vi "Process 4 Page.vi"() -> ()   [LabVIEW 2019]
uses:
  <vilib>/NI/Current Value Table/Type Defs/Single Tag.ctl
  <vilib>/NI/Current Value Table/Type Defs/Data Types.ctl
  <vilib>/NI/STM/TCP/Read Meta Data (TCP Ref).vi
  <vilib>/NI/STM/TCP/Get Connection Reference (TCP).vi
  <vilib>/NI/AMC/Read Termination Message.vi
  <vilib>/NI/AMC/Create Single Message.vi
  <vilib>/NI/AMC/Update Message Routing Info.vi
  <vilib>/NI/STM/TCP/Read Meta Data (TCP Clst).vi
  <vilib>/NI/AMC/Globals.vi
  <vilib>/NI/STM/TCP/Write Message (TCP).vi
  <vilib>/NI/AMC/Send Message.vi
  <vilib>/NI/AMC/AMC.lvlib
  <vilib>/NI/STM/NI STM.lvlib
  <vilib>/NI/Current Value Table/Current Value Table.lvlib
panel:
  in  "Sulfuric Add Volume":dbl min=0.0 max=500.0 step=0.25
  in  "Add Sulfuric":bool
  out "Di Add Pipe 2":bool
  out "Di Water Elbow 2":bool
  out "Liters DI Added 2":dbl caption="Liters Sulfuric Added" format="%.1f"
  out "Sulfuric Flow Rate":dbl(knob) scale=0.0..75.0
  out "Boolean 6":bool
  out "Boolean 5":bool
  in  "Pump Speed 4":dbl=5.0 caption="Pump Speed" min=5.0 max=100.0 step=0.5
  out "RPM":dbl(knob) scale=0.0..3500.0
  out "DI Flow Rate":dbl(knob) scale=0.0..75.0
  out "SG":dbl format="%.4g"
  in  "Bath SG":dbl=1.8 min=0.9 max=1.8 step=0.0025 format="%.4g"
  out "Recirc Elbow":bool
  out "Di Add Pipe":bool
  out "Di Water Elbow":bool
  out "Liters DI Added 1":dbl caption="Liters DI Added" format="%.1f"
  in  "DI Add Volume 1":dbl caption="DI Add Volume" min=0.0 max=500.0 step=0.25
  in  "Add DI water 1":bool caption="Add DI Water"
  in  "Drain System to Tree 1":bool caption="Drain System to Tree"
  in  "Enable Main Pump":bool
  out "Sump Return":bool
  out "PipeFromPmp":bool
  out "Proc4MainPumpInd 2":bool
  out "Tank 2":dbl(slide) caption="Tank" scale=0.0..1000.0
  out "Run Enabled":bool
  in  "Dosing":bool
  in  "Mixing Tank":bool
  in  "Process 3":bool
  in  "Process 2":bool
  in  "Process 1":bool
  out "status":string
  in  "Home Btn":bool
  in  "Facilities Btn":bool
  # "%"
  # "T 340"
  # "L"
  # "@"
  # "L"
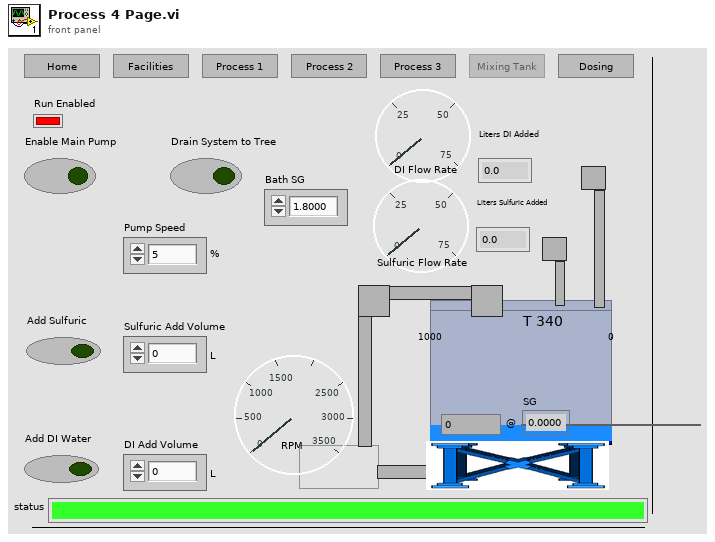
[diagram p1: front panel]
types:
  T1 = typedef "Current Value Table.lvlib/Single Tag.ctl" = cluster{"Data Type":T2, "Name":string, "Value":string, "Description":string}
  T2 = typedef "Current Value Table.lvlib/Data Types.ctl" = enum16{"Double", "Single", "I64", "I32", "I16", "I8", "U64", "U32", "U16", "U8", "String", "Boolean", "Array of U8", "Array of U16", "Array of U32", "Array of U64", "Array of I64", "Array of I32", "Array of I16", "Array of I8", "Array of Double", "Array of Single", "Array of Boolean", "Array of String"}
  T3 = typedef "AMC.lvlib/Message Queue.ctl" = refnum<queue>
  T4 = typedef "NI STM.lvlib/TCP Connection Info.ctl" = cluster{"connection ID":refnum<k5>, "meta data":T5[]}
  T5 = typedef "NI STM.lvlib/MetaDataElement.ctl" = string
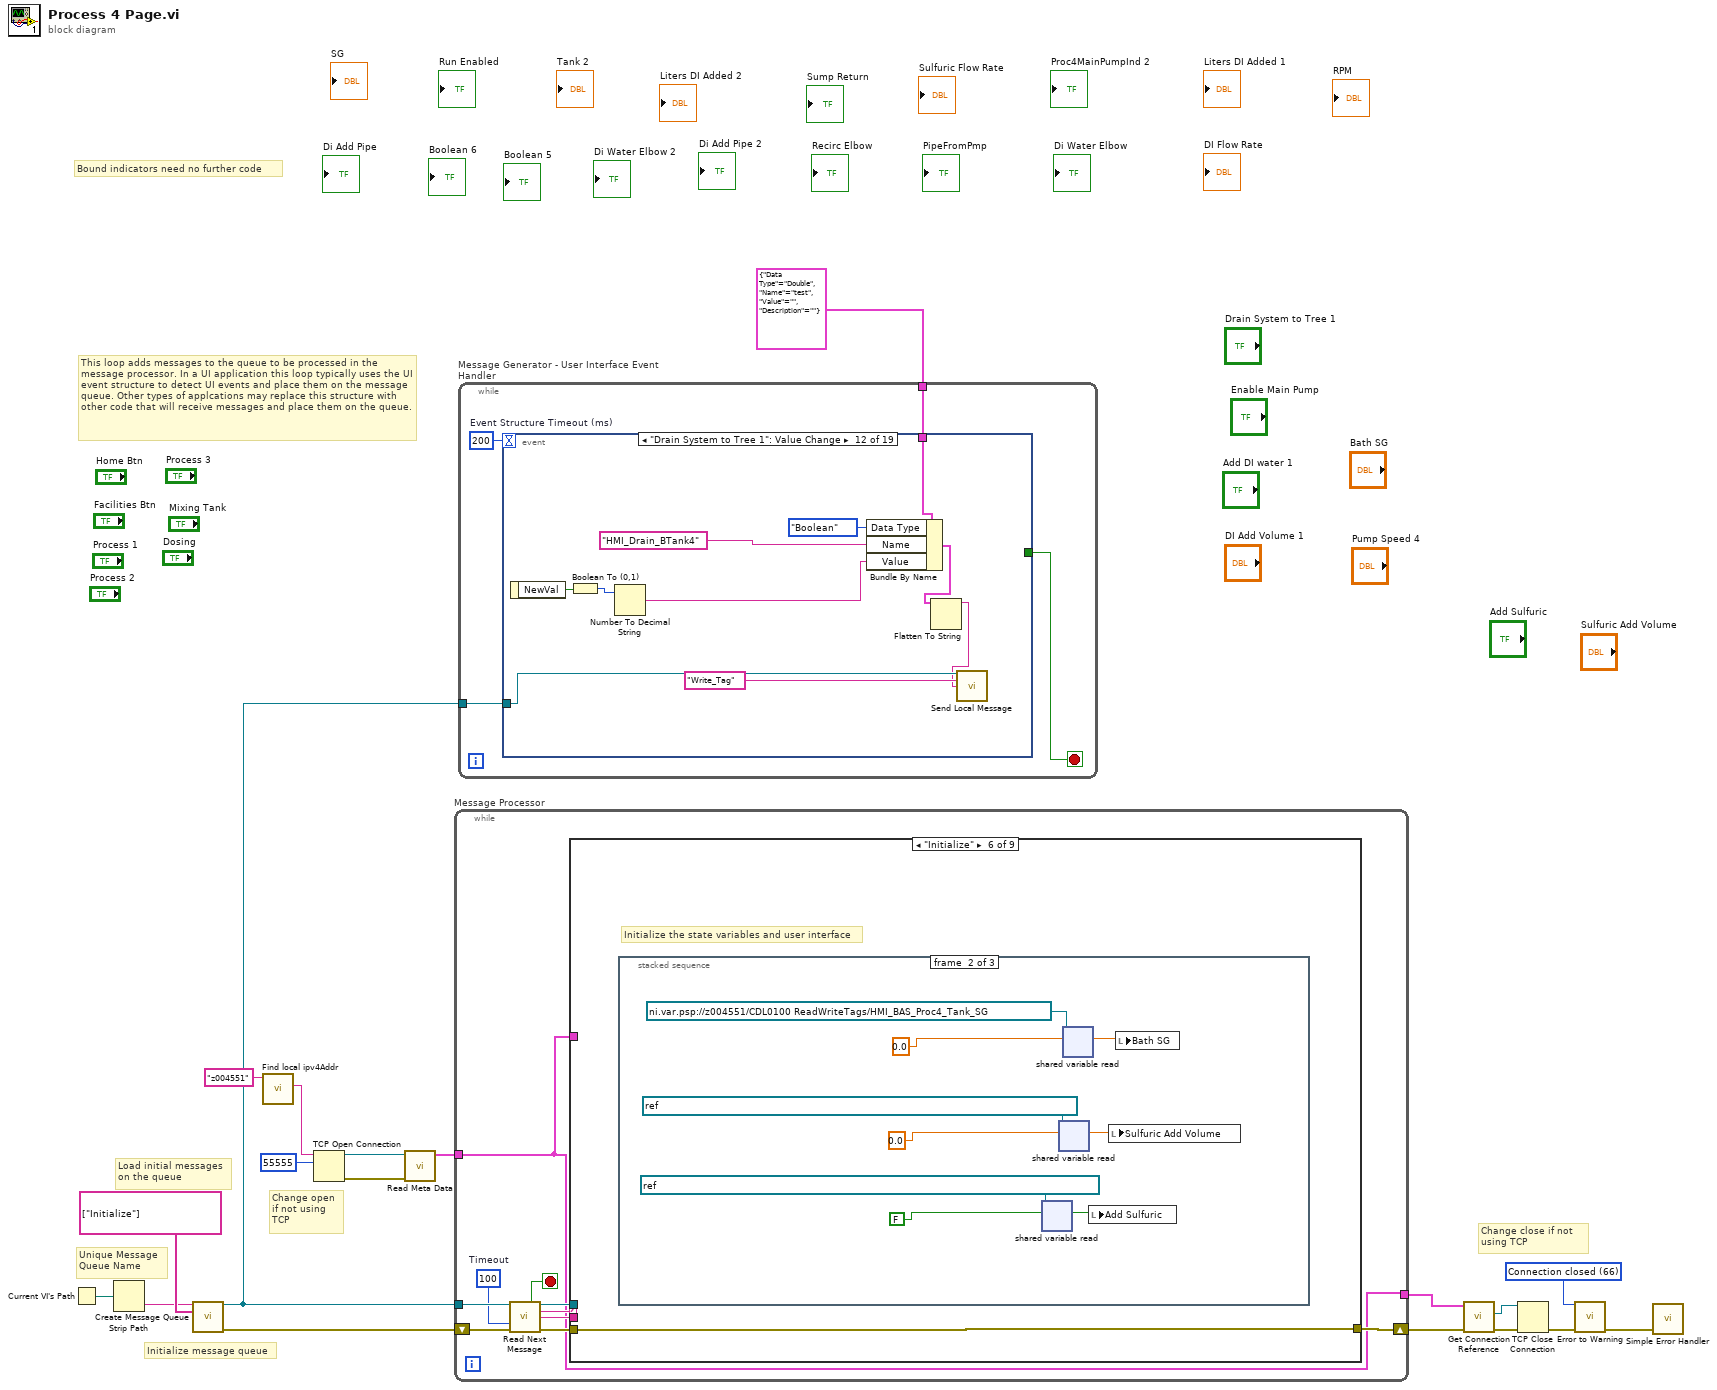
[diagram p0: block diagram]
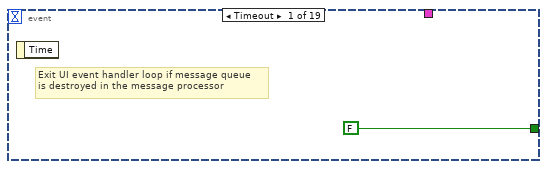
[diagram p2: hidden frame]
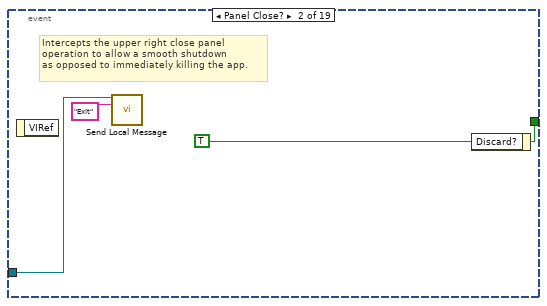
[diagram p3: hidden frame]
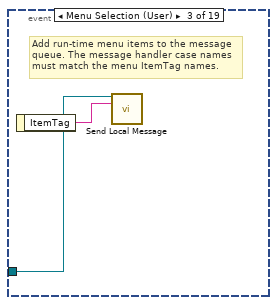
[diagram p4: hidden frame]
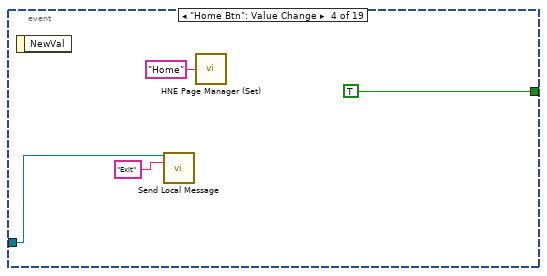
[diagram p5: hidden frame]
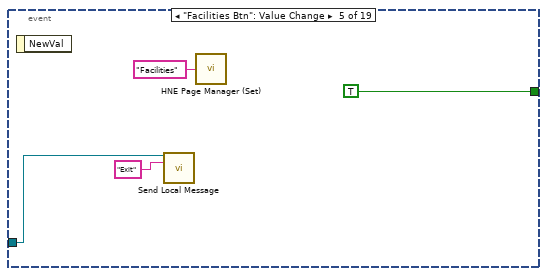
[diagram p6: hidden frame]
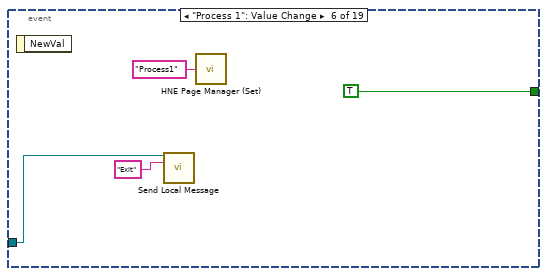
[diagram p7: hidden frame]
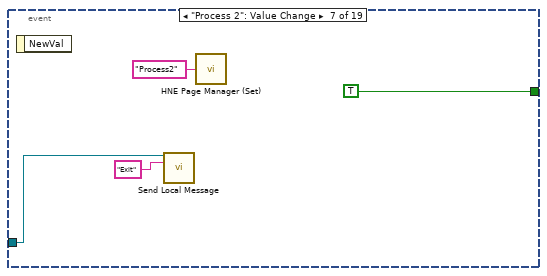
[diagram p8: hidden frame]
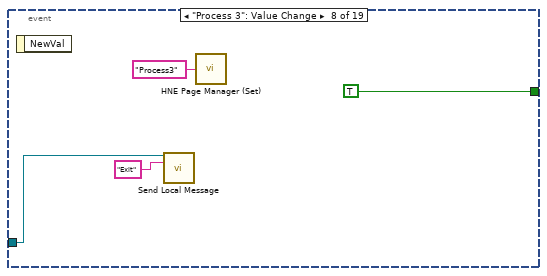
[diagram p9: hidden frame]
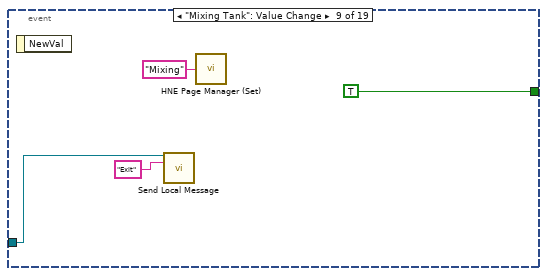
[diagram p10: hidden frame]
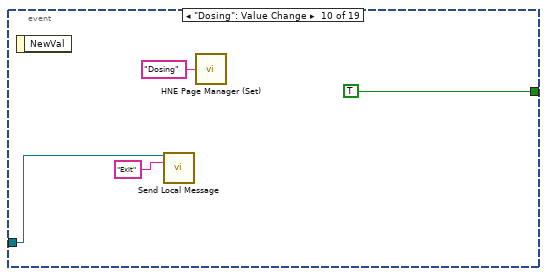
[diagram p11: hidden frame]
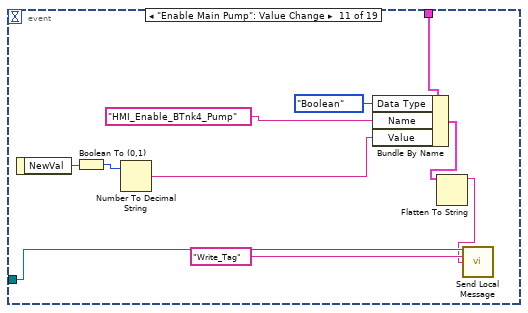
[diagram p12: hidden frame]
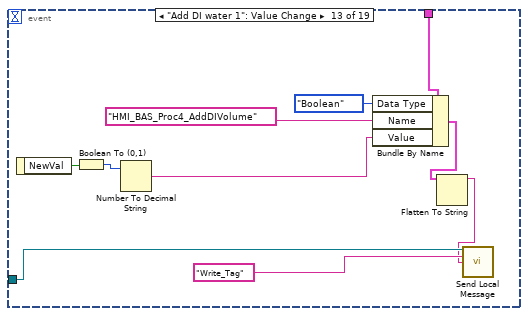
[diagram p13: hidden frame]
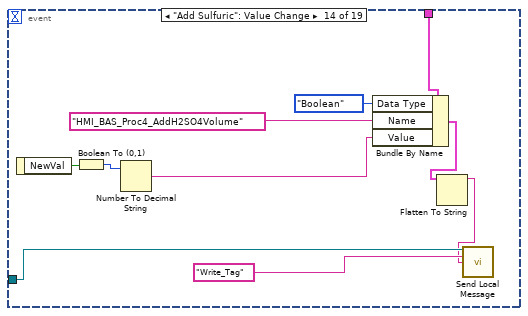
[diagram p14: hidden frame]
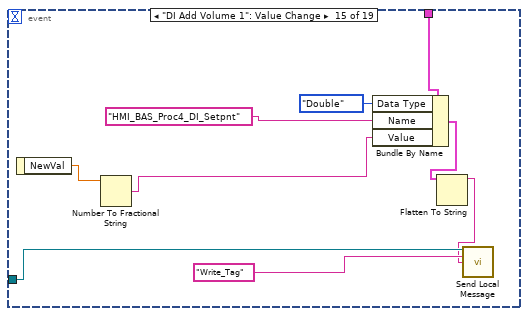
[diagram p15: hidden frame]
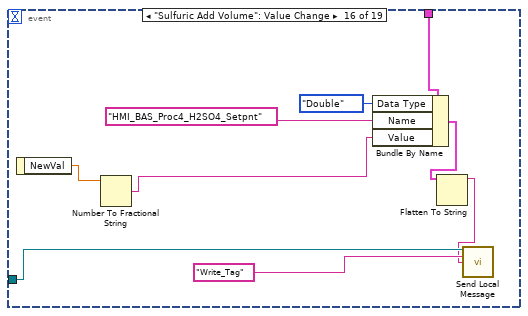
[diagram p16: hidden frame]
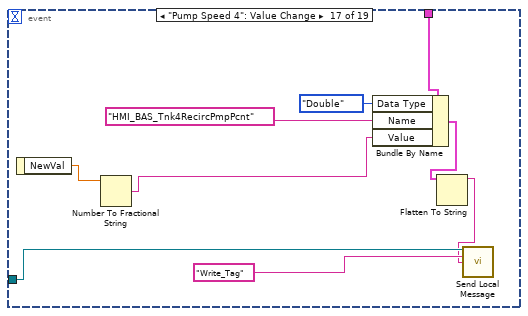
[diagram p17: hidden frame]
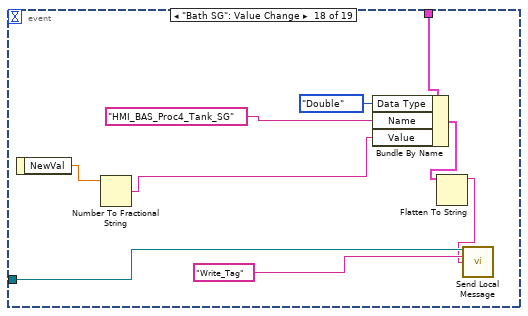
[diagram p18: hidden frame]
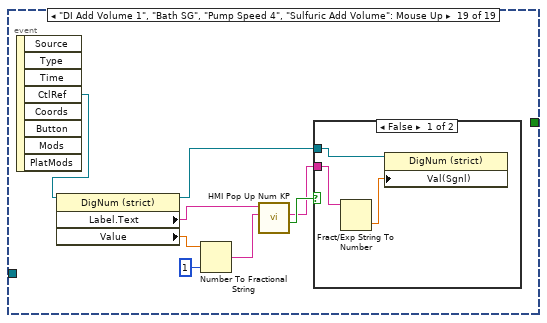
[diagram p19: hidden frame]
diagram:
  w8 = 66 items=["No Error", "Argument Error", "Memory Full", "Out of Zone", "End of File", "File Already Open", "Generic File IO Error", "File Not Found", "File Permission Error", "Disk Full", "Duplicate Path", "Too Many Files Open", "Not Enabled", "Resource File Not Found", "Cannot Add Resource", "Resource Not Found", "Image Not Found", "Image Memory Error", "Pen Does Not Exist", "Config Bad Type", "Config Token Not Found", "Config Parse Error", "Config Memory Error", "Bad External Code Format", "Bad External Code Offset", "External Code Not Present", "Null Window", "Destroy Window Mixup", "Null Menu", "Print Aborted", "Bad Print Record", "Print Driver Error", "Windows Error During Print", "Memory Error During Print", "Print Dialog Error", "Generic Print Error", "Invalid Device Refnum", "Device Not Found", "Device Parameter Error", "Device Unit Error", "Can't Open Device", "Device Call Aborted", "Generic Error", "Cancelled By User", "Object ID Too Low", "Object ID Too High", "Object Not In Heap", "Unknown Heap", "Bad DefProc ID", "DefProc Not In Table", "Message Out Of Range", "Null Method", "Unknown Message", "Manager Call Not Supported", "Bad address", "Connection In progress", "Connection timed out", "Connection is already in progress", "Network attribute not supported", "Network error", "Address in use", "System out of memory", "Connection aborted", "Connection refused", "Connection is not connected", "Connection is already connected", "Connection closed", "Initialize error (interapplication manager)", "Bad occurrence", "Wait on unbound occurrence handler", "Occurrence queue overflow", "Bad path", "Semaphore not signaled", "Unrecognized type (interapplication manager)"] ("1st Error to Convert")
  # "Bound indicators need no further code"
  # "Change close if not using TCP"
  # "Change open if not using TCP"
  # "This loop adds messages to the queue to be processed in the message processor. In a UI application this loop typically uses the UI event structure to detect UI events and place them on the message queue. Other types of applcations may replace this structure with other code that will receive messages and place them on the queue."
  # "Initialize message queue"
  # "Unique Message\nQueue Name"
  # "Load initial messages\non the queue"
  n1 = Current VI's Path() -> (path=w15:path)
  n2 = Strip Path(path=w15) -> (name=w18:string)  [unwired: 1 out]
  n3 = call <vilib>:"Create Message Queue.vi"("message queue name"=w18, "initial message names"=string[] ["Initialize"]) -> ("message queue out"=w17:T3, "error out"=w16:errorcluster)  [unwired: 12 in]
  n4 = call "Find local ipv4Addr.vi"("MachineToFind"="z004551") -> ("name"=w11:string)  [unwired: 9 in, 1 out]
  n5 = TCP Open Connection(address=w11, remote port or service name=u16 55555 ("remote port")) -> (connection ID=w13:refnum<k5>, error out=w12:errorcluster)  [unwired: 1 in, 2 out]
  n6 = call-poly <vilib>:"Read Meta Data.vi"("error in"=w12, "connection ID"=w13) -> ("connection info out"=w3:T4)  [unwired: 7 in, 2 out]
  n7 = while "Message Processor" {
    shift-left: w16 -> [w25]
    shift-right: [w29] -> w4
    tunnel: w17 -> [w26]
    tunnel: [w20] -> w2
    tunnel: w3 -> [w20]
    stop <- w28 stop-if-true
    w21 = 100  # Timeout
    n8 = call <vilib>:"Read Next Message.vi"("message queue in"=w26, "timeout (1 ms)"=w21, "error in"=w25) -> ("exit process?"=w28:bool, "message queue out"=w27:T3, "message name"=w23:string, "message value"=w22:string, "error out"=w24:errorcluster)  [unwired: 5 in, 3 out]
    n9 = case shown="\"Initialize\"" w23 {
      selector: w23 -> [_ _ w56 _ _ _ _ _ _]
      tunnel: w27 -> [_ _ _ _ _ _ w90 _ _]
      tunnel: w24 -> [w30 w32 w57 w58 w60 w61 w91 w93 w95]
      tunnel: [w30 w32 w57 errorcluster {"status"=FALSE, "code"=0, "source"=""} ("error out") w60 w61 w89 w93 w94] -> w29
      tunnel: w22 -> [_ _ _ _ _ _ _ _ w96]
      tunnel: w20 -> [_ _ _ _ _ _ _ _ w97]
      frame "---------- Framework Operations ----------" {
        # "Dummy case to add a seperator in the Case Structure menu"
      }
      frame "", "Idle" {
        # "Idle Case - this case is called after a Timeout on the Get Next Message from Queue VI, if no new messages are present on the queue. This case can be used for housekeeping tasks such as updating the UI."
        n10 = stacked-sequence {
          frame #0 {
            # "Other HMI changed state - align"
            n11 = shared-variable-read(refnum<k21> "ni.var.psp://z004551/CDL0100 ReadWriteTags/HMI_Enable_BTnk4_Pump" ("shared variable refnum in"), FALSE ("data type")) -> (w33:bool)  [unwired: 1 in, 3 out]
            n12 = call <userlib>:"Boolean Trigger__ogtk.vi"("Boolean Input"=w33) -> ("Rising Edge"=w38:bool, "Falling Edge"=w37:bool)  [unwired: 1 in]
            n13 = Or(x=w38, y=w37) -> (x .or. y?=w36:bool)
            n14 = case shown="True" w36 {
              tunnel: w33 -> [_ w39]
              frame False {
              }
              frame True {
                n15 = local write "Enable Main Pump"(w39) -> ()
              }
            }
          }
          frame #1 {
            n16 = shared-variable-read(refnum<k21> "ni.var.psp://z004551/CDL0100 ReadWriteTags/HMI_BAS_Proc4_AddDIVolume" ("shared variable refnum in"), FALSE) -> (w45:bool)  [unwired: 1 in, 3 out]
            n17 = shared-variable-read(refnum<k21> "ni.var.psp://z004551/CDL0100 ReadWriteTags/HMI_BAS_Proc4_AddH2SO4Volume" ("shared variable refnum in"), FALSE) -> (w41:bool)  [unwired: 1 in, 3 out]
            n18 = call <userlib>:"Boolean Trigger__ogtk.vi"("Boolean Input"=w45) -> ("Falling Edge"=w44:bool)  [unwired: 1 in, 1 out]
            n19 = call <userlib>:"Boolean Trigger__ogtk.vi"("Boolean Input"=w41) -> ("Falling Edge"=w40:bool)  [unwired: 1 in, 1 out]
            n20 = case shown="True" w40 {
              frame False {
              }
              frame True {
                n21 = local write "Add Sulfuric"(FALSE) -> ()
              }
            }
            n22 = case shown="True" w44 {
              frame False {
              }
              frame True {
                n23 = local write "Add DI water 1"(FALSE) -> ()
              }
            }
          }
          frame #2 {
            n24 = control-ref of="Enable Main Pump"() -> (w50:refnum<vi>)
            n25 = control-ref of="Drain System to Tree 1"() -> (w52:refnum<vi>)
            n26 = call "GrayOutButtonFromPSPVar.vi"("shared variable refnum in"=refnum<k21> "ni.var.psp://z004551/CDL0100 ReadWriteTags/HMI_Drain_BTank4", "Boolean in"=w50) -> ()  [unwired: 10 in]
            n27 = call "GrayOutButtonFromPSPVar.vi"("shared variable refnum in"=refnum<k21> "ni.var.psp://z004551/CDL0100 ReadWriteTags/HMI_Enable_BTnk4_Pump", "Boolean in"=w52) -> ()  [unwired: 10 in]
          }
        }
        n28 = control-ref of="status"() -> (w31:refnum<vi>)
        n29 = call <userlib>:"TAE Format Alarm Ticker.vi"("Alarm Ticker Ref"=w31) -> ()  [unwired: 15 in]
      }
      frame "Missing Message Handler", Default {
        # "Call this case if a message is received that is not handled \nby any other case. Typically this is a programming error\nas a result of a typo or unhandled message/missing message handler."
        n30 = Format Into String(format string="DevError: Missing message handler for '%s\" message." ("message"), w56) -> (resulting string=w54:string)  [unwired: 2 in, 1 out]
        n31 = One Button Dialog(message=w54) -> ()  [unwired: 2 out]
      }
      frame "Error" {
        # "General Error Case - this case is called if an error is passed using the error cluster below. Typically most new errors should be handed in each individual case and not passed in the rror cluster. If necessary a custom error handler case should be added and called from other cases."
        n32 = call <vilib>:"Simple Error Handler.vi"("error in (no error)"=w58) -> ()  [unwired: 1 in, 8 out]
      }
      frame "---------- Generic Operations ----------" {
        # "Dummy case to add a seperator in the Case Structure menu"
      }
      frame "Initialize" {
        # "Initialize the state variables and user interface"
        n33 = stacked-sequence {
          frame #0 {
            n34 = shared-variable-read(refnum<k21> "ni.var.psp://z004551/CDL0100 ReadWriteTags/HMI_Drain_BTank4" ("shared variable refnum in"), FALSE) -> (w68:bool)  [unwired: 1 in, 3 out]
            n35 = shared-variable-read(refnum<k21> "ni.var.psp://z004551/CDL0100 ReadWriteTags/HMI_BAS_Proc4_AddDIVolume" ("shared variable refnum in"), FALSE) -> (w65:bool)  [unwired: 1 in, 3 out]
            n36 = shared-variable-read(refnum<k21> "ni.var.psp://z004551/CDL0100 ReadWriteTags/HMI_Enable_BTnk4_Pump" ("shared variable refnum in"), FALSE) -> (w71:bool)  [unwired: 1 in, 3 out]
            n37 = shared-variable-read(refnum<k21> "ni.var.psp://z004551/CDL0100 ReadWriteTags/HMI_BAS_Proc4_DI_Setpnt" ("shared variable refnum in"), 0.0) -> (w62:dbl)  [unwired: 1 in, 3 out]
            n38 = local write "Drain System to Tree 1"(w68) -> ()
            n39 = local write "Add DI water 1"(w65) -> ()
            n40 = local write "Enable Main Pump"(w71) -> ()
            n41 = local write "DI Add Volume 1"(w62) -> ()
          }
          frame #1 {
            n42 = shared-variable-read(refnum<k21> "ni.var.psp://z004551/CDL0100 ReadWriteTags/HMI_BAS_Proc4_AddH2SO4Volume" ("shared variable refnum in"), FALSE) -> (w74:bool)  [unwired: 1 in, 3 out]
            n43 = shared-variable-read(refnum<k21> "ni.var.psp://z004551/CDL0100 ReadWriteTags/HMI_BAS_Proc4_H2SO4_Setpnt" ("shared variable refnum in"), 0.0) -> (w77:dbl)  [unwired: 1 in, 3 out]
            n44 = shared-variable-read(refnum<k21> "ni.var.psp://z004551/CDL0100 ReadWriteTags/HMI_BAS_Proc4_Tank_SG" ("shared variable refnum in"), 0.0) -> (w80:dbl)  [unwired: 1 in, 3 out]
            n45 = local write "Add Sulfuric"(w74) -> ()
            n46 = local write "Sulfuric Add Volume"(w77) -> ()
            n47 = local write "Bath SG"(w80) -> ()
          }
          frame #2 {
            n48 = shared-variable-read(refnum<k21> "ni.var.psp://z004551/CDL0100 ReadTags/BAS_Proc4_DI_FlowRate" ("shared variable refnum in"), 0.0) -> (w86:dbl)  [unwired: 1 in, 3 out]
            n49 = shared-variable-read(refnum<k21> "ni.var.psp://z004551/CDL0100 ReadWriteTags/HMI_BAS_Tnk4RecircPmpPcnt" ("shared variable refnum in"), 0.0) -> (w83:dbl)  [unwired: 1 in, 3 out]
            n50 = local write "Pump Speed 4"(w83) -> ()
            n51 = local write "DI Flow Rate"(w86) -> ()
          }
        }
      }
      frame "Exit" {
        # "Destroy message queue >> this will halt the UI event handler loop"
        # "Stop the VI\n>> Perform any cleanup tasks in this message case.\n>> Clear display before closing."
        n52 = call <vilib>:"Destroy Message Queue.vi"("message queue in"=w90, "error in"=w91) -> ("error out"=w89:errorcluster)  [unwired: 11 in, 2 out]
        n53 = local write "status"("" ("Status")) -> ()
      }
      frame "---------- Application Operations ----------" {
        # "Dummy case to add a seperator in the Case Structure menu"
      }
      frame "Write_Tag" {
        n54 = call-poly <vilib>:"Write Message.vi"("error in"=w95, "data"=w96, "name"="WriteTag", "connection info in"=w97) -> ("error out"=w94:errorcluster)  [unwired: 6 in, 1 out]
      }
    }
  }
  n55 = while "Message Generator - User Interface Event Handler" {
    tunnel: w17 -> [w100]
    tunnel: T1 {"Data Type"=enum."Double", "Name"="test", "Value"="", "Description"=""} ("Tag") -> [w99]
    stop <- w101 stop-if-true
    w102 = 200  # Event Structure Timeout (ms)
    n56 = event shown="[11] \"Drain System to Tree 1\": Value Change" {
      selector: _ -> [_ _ _ _ _ _ _ _ _ _ _ _ _ _ _ _ _ _ _]
      dyn-events: _ -> [_ _ _ _ _ _ _ _ _ _ _ _ _ _ _ _ _ _ _]
      timeout: w102 -> [_ _ _ _ _ _ _ _ _ _ _ _ _ _ _ _ _ _ _]
      tunnel: [FALSE ("Discard?") w106 _ TRUE ("Discard?") TRUE ("Discard?") TRUE ("Discard?") TRUE ("Discard?") TRUE ("Discard?") TRUE ("Discard?") TRUE ("Discard?") _ _ _ _ _ _ _ _ _] -> w101
      tunnel: w100 -> [_ w104 w107 w109 w113 w117 w121 w125 w129 w133 w139 w149 w159 w169 w181 w190 w199 w208 _]
      tunnel: w99 -> [_ _ _ _ _ _ _ _ _ _ w144 w154 w164 w174 w185 w194 w203 w212 _]
      event Timeout {
        # "Exit UI event handler loop if message queue\nis destroyed in the message processor"
        n57 = event-data() -> ()  [unwired: 2 out]
      }
      event Panel Close? {
        w106 = TRUE ("Discard?")
        # "Intercepts the upper right close panel\noperation to allow a smooth shutdown\nas opposed to immediately killing the app."
        n58 = event-data() -> ()  [unwired: 2 out]
        n59 = call <vilib>:"Send Local Message.vi"("message queue in"=w104, "message name"="Exit") -> ()  [unwired: 11 in, 3 out]
        n60 = event-data("Discard?"=w106) -> ()  [unwired: 1 in, 1 out]
      }
      event Menu Selection (User) {
        # "Add run-time menu items to the message\nqueue. The message handler case names must match the menu ItemTag names."
        n61 = event-data() -> ("ItemTag"=w108:string)  [unwired: 1 out]
        n62 = call <vilib>:"Send Local Message.vi"("message queue in"=w107, "message name"=w108) -> ()  [unwired: 11 in, 3 out]
      }
      event "Home Btn": Value Change {
        n63 = event-data() -> ()  [unwired: 2 out]
        n64 = call <vilib>:"Send Local Message.vi"("message queue in"=w109, "message name"="Exit") -> ()  [unwired: 11 in, 3 out]
        n65 = call <userlib>:"HNE Page Manager (Set).vi"("Next Page"="Home") -> ()  [unwired: 4 in, 1 out]
      }
      event "Facilities Btn": Value Change {
        n66 = event-data() -> ()  [unwired: 2 out]
        n67 = call <vilib>:"Send Local Message.vi"("message queue in"=w113, "message name"="Exit") -> ()  [unwired: 11 in, 3 out]
        n68 = call <userlib>:"HNE Page Manager (Set).vi"("Next Page"="Facilities") -> ()  [unwired: 4 in, 1 out]
      }
      event "Process 1": Value Change {
        n69 = event-data() -> ()  [unwired: 2 out]
        n70 = call <vilib>:"Send Local Message.vi"("message queue in"=w117, "message name"="Exit") -> ()  [unwired: 11 in, 3 out]
        n71 = call <userlib>:"HNE Page Manager (Set).vi"("Next Page"="Process1") -> ()  [unwired: 4 in, 1 out]
      }
      event "Process 2": Value Change {
        n72 = event-data() -> ()  [unwired: 2 out]
        n73 = call <vilib>:"Send Local Message.vi"("message queue in"=w121, "message name"="Exit") -> ()  [unwired: 11 in, 3 out]
        n74 = call <userlib>:"HNE Page Manager (Set).vi"("Next Page"="Process2") -> ()  [unwired: 4 in, 1 out]
      }
      event "Process 3": Value Change {
        n75 = event-data() -> ()  [unwired: 2 out]
        n76 = call <vilib>:"Send Local Message.vi"("message queue in"=w125, "message name"="Exit") -> ()  [unwired: 11 in, 3 out]
        n77 = call <userlib>:"HNE Page Manager (Set).vi"("Next Page"="Process3") -> ()  [unwired: 4 in, 1 out]
      }
      event "Mixing Tank": Value Change {
        n78 = event-data() -> ()  [unwired: 2 out]
        n79 = call <vilib>:"Send Local Message.vi"("message queue in"=w129, "message name"="Exit") -> ()  [unwired: 11 in, 3 out]
        n80 = call <userlib>:"HNE Page Manager (Set).vi"("Next Page"="Mixing") -> ()  [unwired: 4 in, 1 out]
      }
      event "Dosing": Value Change {
        n81 = event-data() -> ()  [unwired: 2 out]
        n82 = call <vilib>:"Send Local Message.vi"("message queue in"=w133, "message name"="Exit") -> ()  [unwired: 11 in, 3 out]
        n83 = call <userlib>:"HNE Page Manager (Set).vi"("Next Page"="Dosing") -> ()  [unwired: 4 in, 1 out]
      }
      event "Enable Main Pump": Value Change {
        n84 = event-data() -> ("NewVal"=w146:bool)  [unwired: 1 out]
        n85 = Boolean To (0,1)(Boolean=w146) -> (0, 1=w145:i16)
        n86 = Number To Decimal String(number=w145) -> (decimal integer string=w141:string)  [unwired: 1 in]
        n87 = Bundle By Name(cluster=w144, "Data Type"=Data_Types."Boolean", "Name"="HMI_Enable_BTnk4_Pump", "Value"=w141) -> (w140:T1)
        n88 = Flatten To String(anything=w140) -> (data string=w137:string)  [unwired: 3 in, 2 out]
        n89 = call <vilib>:"Send Local Message.vi"("message queue in"=w139, "message name"="Write_Tag", "message value"=w137) -> ()  [unwired: 10 in, 3 out]
      }
      event "Drain System to Tree 1": Value Change {
        n90 = event-data() -> ("NewVal"=w156:bool)  [unwired: 1 out]
        n91 = Boolean To (0,1)(Boolean=w156) -> (0, 1=w155:i16)
        n92 = Number To Decimal String(number=w155) -> (decimal integer string=w151:string)  [unwired: 1 in]
        n93 = Bundle By Name(cluster=w154, "Data Type"=Data_Types."Boolean", "Name"="HMI_Drain_BTank4", "Value"=w151) -> (w150:T1)
        n94 = Flatten To String(anything=w150) -> (data string=w147:string)  [unwired: 3 in, 2 out]
        n95 = call <vilib>:"Send Local Message.vi"("message queue in"=w149, "message name"="Write_Tag", "message value"=w147) -> ()  [unwired: 10 in, 3 out]
      }
      event "Add DI water 1": Value Change {
        n96 = event-data() -> ("NewVal"=w166:bool)  [unwired: 1 out]
        n97 = Boolean To (0,1)(Boolean=w166) -> (0, 1=w165:i16)
        n98 = Number To Decimal String(number=w165) -> (decimal integer string=w161:string)  [unwired: 1 in]
        n99 = Bundle By Name(cluster=w164, "Data Type"=Data_Types."Boolean", "Name"="HMI_BAS_Proc4_AddDIVolume", "Value"=w161) -> (w160:T1)
        n100 = Flatten To String(anything=w160) -> (data string=w157:string)  [unwired: 3 in, 2 out]
        n101 = call <vilib>:"Send Local Message.vi"("message queue in"=w159, "message name"="Write_Tag", "message value"=w157) -> ()  [unwired: 10 in, 3 out]
      }
      event "Add Sulfuric": Value Change {
        n102 = event-data() -> ("NewVal"=w176:bool)  [unwired: 1 out]
        n103 = Boolean To (0,1)(Boolean=w176) -> (0, 1=w175:i16)
        n104 = Number To Decimal String(number=w175) -> (decimal integer string=w171:string)  [unwired: 1 in]
        n105 = Bundle By Name(cluster=w174, "Data Type"=Data_Types."Boolean", "Name"="HMI_BAS_Proc4_AddH2SO4Volume", "Value"=w171) -> (w170:T1)
        n106 = Flatten To String(anything=w170) -> (data string=w167:string)  [unwired: 3 in, 2 out]
        n107 = call <vilib>:"Send Local Message.vi"("message queue in"=w169, "message name"="Write_Tag", "message value"=w167) -> ()  [unwired: 10 in, 3 out]
      }
      event "DI Add Volume 1": Value Change {
        n108 = event-data() -> ("NewVal"=w178:dbl)  [unwired: 1 out]
        n109 = Number To Fractional String(number=w178) -> (F-format string=w177:string)  [unwired: 3 in]
        n110 = Bundle By Name(cluster=w185, "Data Type"=Data_Types."Double", "Name"="HMI_BAS_Proc4_DI_Setpnt", "Value"=w177) -> (w182:T1)
        n111 = Flatten To String(anything=w182) -> (data string=w179:string)  [unwired: 3 in, 2 out]
        n112 = call <vilib>:"Send Local Message.vi"("message queue in"=w181, "message name"="Write_Tag", "message value"=w179) -> ()  [unwired: 10 in, 3 out]
      }
      event "Sulfuric Add Volume": Value Change {
        n113 = event-data() -> ("NewVal"=w187:dbl)  [unwired: 1 out]
        n114 = Number To Fractional String(number=w187) -> (F-format string=w186:string)  [unwired: 3 in]
        n115 = Bundle By Name(cluster=w194, "Data Type"=Data_Types."Double", "Name"="HMI_BAS_Proc4_H2SO4_Setpnt", "Value"=w186) -> (w191:T1)
        n116 = Flatten To String(anything=w191) -> (data string=w188:string)  [unwired: 3 in, 2 out]
        n117 = call <vilib>:"Send Local Message.vi"("message queue in"=w190, "message name"="Write_Tag", "message value"=w188) -> ()  [unwired: 10 in, 3 out]
      }
      event "Pump Speed 4": Value Change {
        n118 = event-data() -> ("NewVal"=w196:dbl)  [unwired: 1 out]
        n119 = Number To Fractional String(number=w196) -> (F-format string=w195:string)  [unwired: 3 in]
        n120 = Bundle By Name(cluster=w203, "Data Type"=Data_Types."Double", "Name"="HMI_BAS_Tnk4RecircPmpPcnt", "Value"=w195) -> (w200:T1)
        n121 = Flatten To String(anything=w200) -> (data string=w197:string)  [unwired: 3 in, 2 out]
        n122 = call <vilib>:"Send Local Message.vi"("message queue in"=w199, "message name"="Write_Tag", "message value"=w197) -> ()  [unwired: 10 in, 3 out]
      }
      event "Bath SG": Value Change {
        n123 = event-data() -> ("NewVal"=w205:dbl)  [unwired: 1 out]
        n124 = Number To Fractional String(number=w205) -> (F-format string=w204:string)  [unwired: 3 in]
        n125 = Bundle By Name(cluster=w212, "Data Type"=Data_Types."Double", "Name"="HMI_BAS_Proc4_Tank_SG", "Value"=w204) -> (w209:T1)
        n126 = Flatten To String(anything=w209) -> (data string=w206:string)  [unwired: 3 in, 2 out]
        n127 = call <vilib>:"Send Local Message.vi"("message queue in"=w208, "message name"="Write_Tag", "message value"=w206) -> ()  [unwired: 10 in, 3 out]
      }
      event "DI Add Volume 1", "Bath SG", "Pump Speed 4", "Sulfuric Add Volume": Mouse Up {
        n128 = event-data() -> ("CtlRef"=w213:refnum<vi>)  [unwired: 8 out]
        n129 = property class="DigNum (strict)"(reference=w213) -> (reference out=w214:refnum<vi>, "Label.Text"=w220:string, "Value"=w219:dbl)  [unwired: 1 in, 1 out]
        n130 = Number To Fractional String(number=w219, precision (6)=i16 1) -> (F-format string=w218:string)  [unwired: 2 in]
        n131 = call <userlib>:"HMI Pop Up Num KP.vi"("String In"=w218, "Message In"=w220) -> ("Canceled"=w216:bool, "String Out"=w215:string)  [unwired: 8 in]
        n132 = case shown="False" w216 {
          tunnel: w215 -> [w222 _]
          tunnel: w214 -> [w223 _]
          frame False {
            n133 = Fract/Exp String To Number(string=w222) -> (number=w221:dbl)  [unwired: 3 in, 1 out]
            n134 = property class="DigNum (strict)"(reference=w223, "Val(Sgnl)"=w221) -> ()  [unwired: 1 in, 2 out]
          }
          frame True {
          }
        }
      }
    }
  }
  n135 = call-poly <vilib>:"Get Connection Reference.vi"("error in"=w4, "connection info in"=w2) -> ("error out"=w7:errorcluster, "connection ID out"=w6:refnum<k5>)  [unwired: 8 out]
  n136 = TCP Close Connection(connection ID=w6, error in (no error)=w7) -> (error out=w9:errorcluster)  [unwired: 2 out]
  n137 = call <vilib>:"Error to Warning.vi"("1st Error to Convert"=w8, "error in"=w9) -> ("warning out"=w5:errorcluster)  [unwired: 3 in, 10 out]
  n138 = call <vilib>:"Simple Error Handler.vi"("error in (no error)"=w5) -> ()  [unwired: 4 in, 5 out]
